vi "Flipper Control Servo.vi"(2 "Frisbee States":T1, 3 "Cannon Position(deg)":dbl, 4 "Enable Stack":bool) -> (0 "Stop Conveyer Belt":bool, 1 "Set Flipper's Servos Angle":i32)   [LabVIEW 2012]
panel:
  # "Flipper Angle"
  # "Cannon Angle"
  # "90"
  # "90-min / 90"
  # "170"
  # "0 / min angle"
  # "90 / min+90"
  # "48.6 => 49"
  # "-min angle / 0"
  # "0"
  # "original angle / \"Cannon Position(deg)\""
  # "FlipperAtPlace is True if the servo is at 0 degrees"
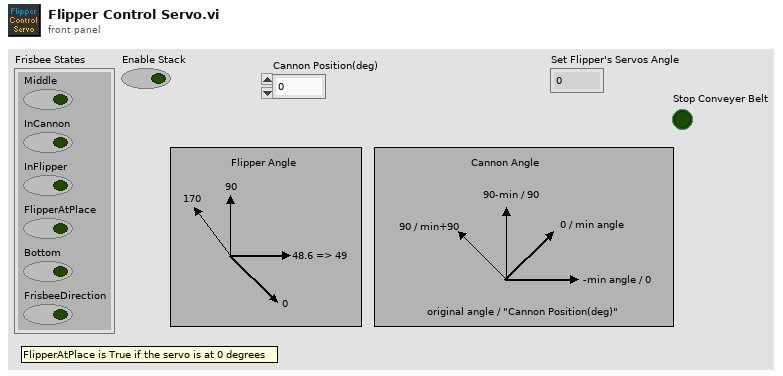
[diagram p1: front panel]
types:
  T1 = cluster{"Middle":bool, "InCannon":bool, "InFlipper":bool, "FlipperAtPlace":bool, "Bottom":bool, "FrisbeeDirection":bool}
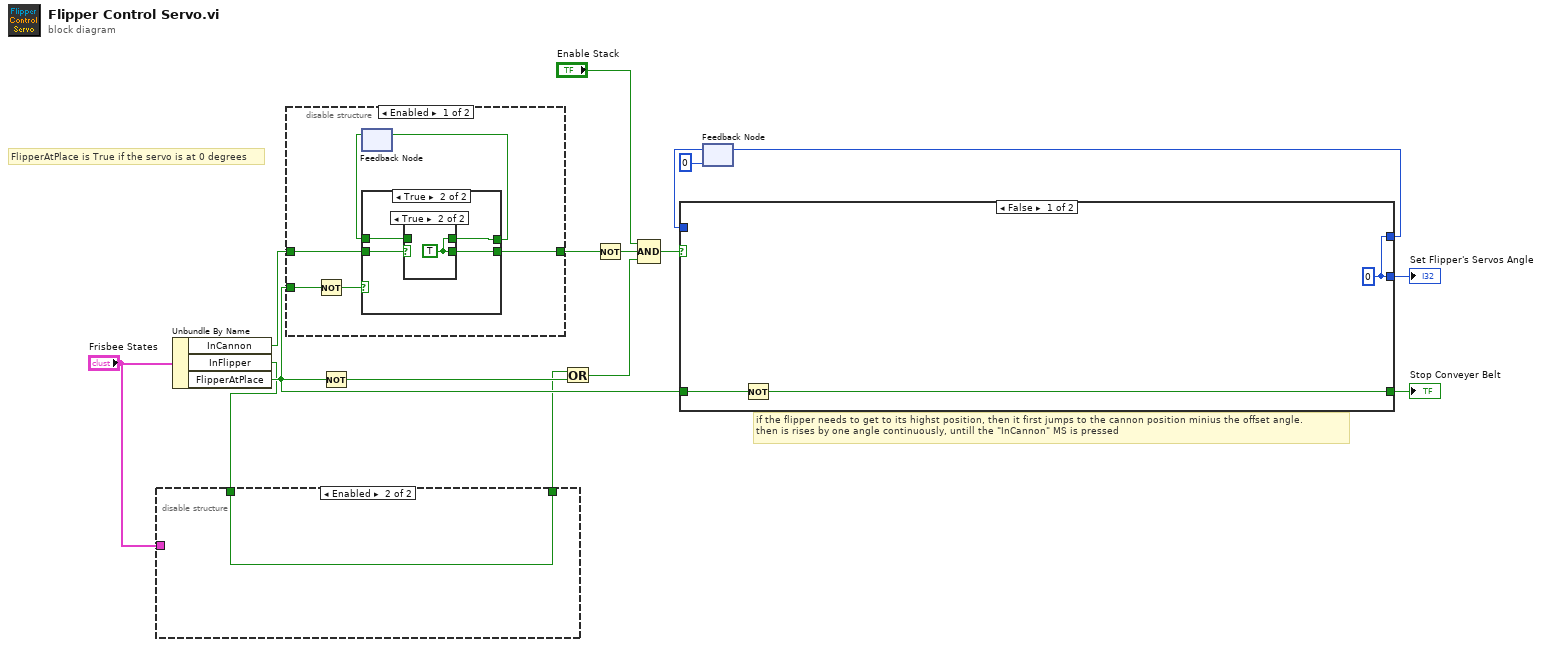
[diagram p0: block diagram]
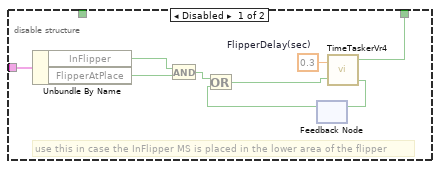
[diagram p2: hidden frame]
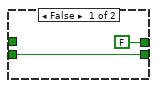
[diagram p3: hidden frame]
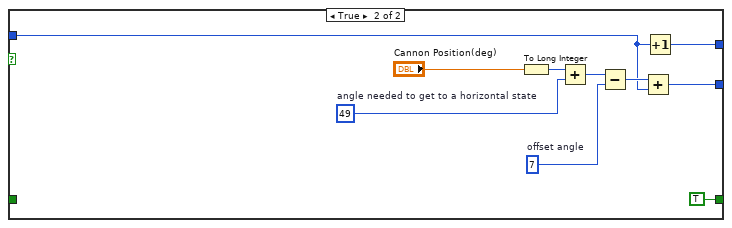
[diagram p6: hidden frame]
diagram:
  # "FlipperAtPlace is True if the servo is at 0 degrees"
  # "if the flipper needs to get to its highst position, then it first jumps to the cannon position minius the offset angle.\nthen is rises by one angle continuously, untill the \"InCannon\" MS is pressed"
  n1 = Unbundle By Name("Frisbee States") -> ("InCannon"=w5:bool, "InFlipper"=w2:bool, "FlipperAtPlace"=w6:bool)
  n2 = disable-structure shown="Enabled" {
    disable-tunnel: "Frisbee States" -> [w25 _]
    disable-tunnel: [w17 w26] -> w1
    disable-tunnel: w2 -> [_ w26]
    frame Disabled {
      w18 = 0.3  # FlipperDelay(sec)
      # "use this in case the InFlipper MS is placed in the lower area of the flipper"
      n3 = Unbundle By Name(w25) -> ("InFlipper"=w20:bool, "FlipperAtPlace"=w19:bool)
      n4 = And(x=w20, y=w19) -> (x .and. y?=w24:bool)
      n5 = feedback #1() -> (w23:bool)  [unwired: 1 in]
      n6 = Or(x=w24, y=w23) -> (x .or. y?=w21:bool)
      n7 = call "TimeTaskerVr4.vi"("Delay(sec)"=w18, "Start Counting?"=w21) -> ("TimePast?"=w17:bool, "Counting?"=w22:bool)  [unwired: 1 out]
      n8 = feedback-in #1(w22) -> ()
    }
    frame Enabled {
    }
  }
  n9 = disable-structure shown="Enabled" {
    disable-tunnel: w6 -> [w29 _]
    disable-tunnel: w5 -> [w28 w41]
    disable-tunnel: [w27 w41] -> w4
    frame Enabled {
      n10 = Not(x=w29) -> (.not. x?=w30:bool)
      n11 = feedback #2() -> (w31:bool)  [unwired: 1 in]
      n12 = case shown="True" w30 {
        tunnel: [w34 w35] -> w27
        tunnel: w28 -> [w34 w38]
        tunnel: [FALSE w37] -> w32
        tunnel: w31 -> [_ w36]
        frame False {
        }
        frame True {
          n13 = case shown="True" w38 {
            tunnel: [w39 w40] -> w37
            tunnel: w36 -> [w39 _]
            tunnel: [w39 w40] -> w35
            frame False {
            }
            frame True {
              w40 = TRUE
            }
          }
        }
      }
      n14 = feedback-in #2(w32) -> ()
    }
    frame Disabled {
      # "use this in case the InCannon MS is\nplaced on the flipper at all time"
    }
  }
  n15 = Not(x=w6) -> (.not. x?=w14:bool)
  n16 = Or(x=w1, y=w14) -> (x .or. y?=w15:bool)
  n17 = Not(x=w4) -> (.not. x?=w16:bool)
  n18 = Compound Arithmetic op=AND("Enable Stack", w16, w15) -> (w13:bool)
  n19 = feedback #3(0) -> (w11:i32)
  n20 = case shown="False" w13 {
    tunnel: [w44 w48] -> w10
    tunnel: [w44 w49] -> w12
    tunnel: w11 -> [_ w47]
    tunnel: [w42 TRUE ("Stop Conveyer Belt")] -> w8
    tunnel: w6 -> [w43 _]
    frame False {
      w44 = 0
      n21 = Not(x=w43) -> (.not. x?=w42:bool)
    }
    frame True {
      w54 = 49  # angle needed to get to a horizontal state
      w52 = 7  # offset angle
      n22 = To Long Integer(number="Cannon Position(deg)") -> (32bit integer=w51:i32)
      n23 = Add(x=w51, y=w54) -> (x+y=w53:i32)
      n24 = Subtract(x=w53, y=w52) -> (x-y=w50:i32)
      n25 = Add(x=w50, y=w47) -> (x+y=w48:i32)
      n26 = Increment(x=w47) -> (x+1=w49:i32)
    }
  }
  "Set Flipper's Servos Angle" <- w10
  "Stop Conveyer Belt" <- w8
  n27 = feedback-in #3(w12) -> ()
